vi "CentralStorage.Exit.vi"(8 "error in (no error)":errorcluster, 11 "CentralStorage in":refnum<class "CentralStorage.lvclass">) -> (0 "error out":errorcluster, 3 "CentralStorage out":refnum<class "CentralStorage.lvclass">)   [LabVIEW 2016, in "CentralStorage.lvclass"]
uses:
  CentralStorage.lvclass
  CentralStorage.lvclass/CentralStorage.ctl
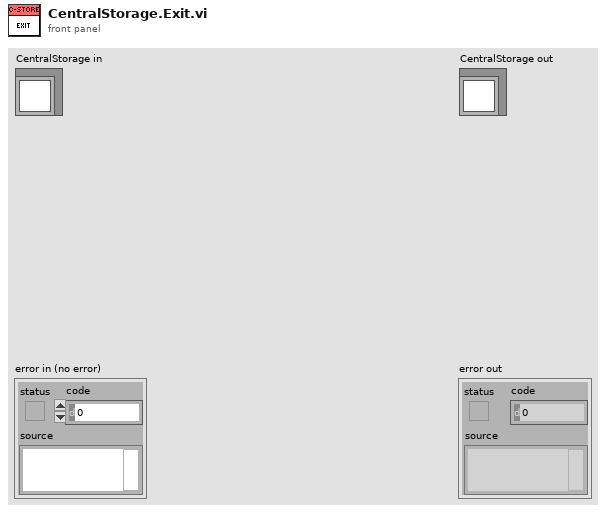
[diagram p1: front panel]
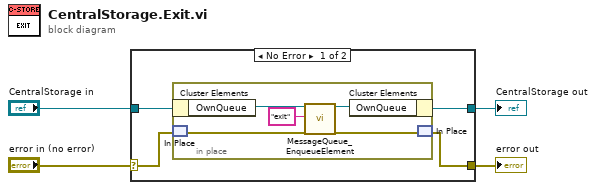
[diagram p0: block diagram]
diagram:
  n1 = case shown="No Error" "error in (no error)" {
    selector: "error in (no error)" -> [w6 w15]
    tunnel: [w5 w15] -> w3
    tunnel: [w7 w14] -> w1
    tunnel: "CentralStorage in" -> [w8 w14]
    frame No Error {
      n2 = in-place {
        n3 = in-place-cluster #1(w8) -> ("OwnQueue"=w13:refnum<queue>)
        n4 = in-place-match #2(w6) -> (w10:errorcluster)
        n5 = call "MessageQueue_EnqueueElement.vi"("QueueIn"=w13, "Message"="exit", "ErrorIn"=w10) -> ("QueueOut"=w12:refnum<queue>, "ErrorOut"=w9:errorcluster)  [unwired: 15 in]
        n6 = in-place-cluster #1("OwnQueue"=w12) -> (w7:refnum<class "CentralStorage.lvclass">)
        n7 = in-place-match #2(w9) -> (w5:errorcluster)
      }
    }
    frame Error {
    }
  }
  "error out" <- w3
  "CentralStorage out" <- w1
